vi "f_drn__v1.vi"(9 "n":ext, 10 "R":ext, 11 "D":ext) -> (3 "出力結果":ext)   [LabVIEW 2020]
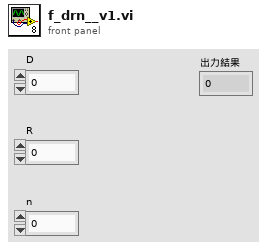
[diagram p1: front panel]
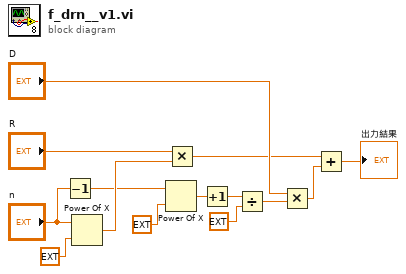
[diagram p0: block diagram]
diagram:
  n1 = Decrement(x="n") -> (x-1=w9:ext)
  n2 = Power Of X(1:ext -1.0, 2:"n") -> (0:w12:ext)
  n3 = Power Of X(1:ext -1.0, 2:w9) -> (0:w8:ext)
  n4 = Multiply(x="R", y=w12) -> (x*y=w2:ext)
  n5 = Increment(x=w8) -> (x+1=w7:ext)
  n6 = Divide(x=w7, y=ext 2.0) -> (x/y=w5:ext)
  n7 = Multiply(x="D", y=w5) -> (x*y=w3:ext)
  n8 = Add(x=w2, y=w3) -> (x+y=→"出力結果":ext)
